vi "State_Machine.vi"(8 "error in (no error)":errorcluster caption="entrée d'erreur (pas d'erreur)", 11 "Wait_CloseFixture en entrée":refnum<class "Put_Weight.lvclass">) -> (0 "error out":errorcluster caption="sortie d'erreur", 2 "Json_String":string, 3 "Wait_CloseFixture en sortie":refnum<class "Put_Weight.lvclass">)   [LabVIEW 2020, in "Library Test.lvlib" / "Put_Weight.lvclass"]
uses:
  Put_Weight.lvclass
  C:/Users/ngarcin/OneDrive - Altyor/Standard TB/Class/Test/Test (Default)/Test (Default).lvclass
  Instrument/Instrument (Default)/Class Instrument (Default).lvclass
  Popup/Class Popup WaitWeight/Class Popup WaitWeight.lvclass
  C:/Users/ngarcin/OneDrive - Altyor/Standard TB/Class/Popup/Class Popup Operator_Validation/Class Popup Operator_Validation (Default)/Class Popup Operator_Validation (Virtual).lvclass
  C:/Users/ngarcin/OneDrive - Altyor/Standard TB/Class/Popup/Class Popup (Main)/Class Popup (Main).lvclass
  Put_Weight.lvclass/Put_Weight.ctl
  Commun VI/Library Commun.lvlib
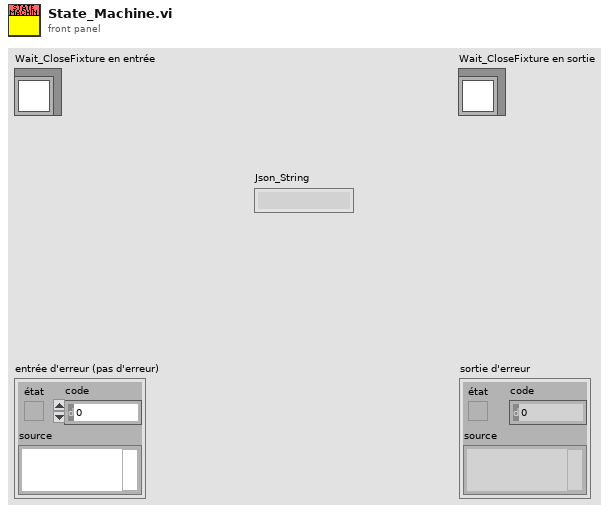
[diagram p1: front panel]
types:
  T1 = cluster{"Instrument":refnum<class "Class Instrument (Default).lvclass">, "Timeout (ms)":u64, "Weight":dbl, "Front":enum16{"Amount", "Descending"}}
  T2 = cluster{"Instrument DIO":refnum<class "Class Instrument (Default).lvclass">, "Valur for test":bool, "Timeout (ms)":u64}
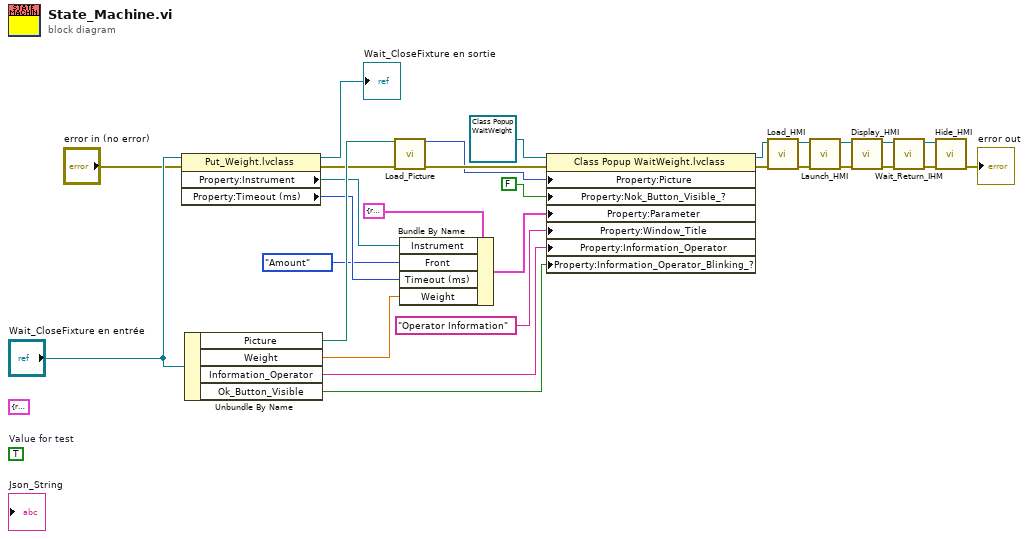
[diagram p0: block diagram]
diagram:
  (unwired) T2 {"Instrument DIO"=refnum, "Valur for test"=FALSE, "Timeout (ms)"=0} ("cluster")
  (unwired) TRUE  # Value for test
  n1 = property class="Put_Weight.lvclass"(reference="Wait_CloseFixture en entrée", error in="error in (no error)") -> (reference out=→"Wait_CloseFixture en sortie":refnum<class "Put_Weight.lvclass">, error out=w6:errorcluster, "Property:Instrument"=w8:refnum<class "Class Instrument (Default).lvclass">, "Property:Timeout (ms)"=w13:u64)
  n2 = Unbundle By Name("Wait_CloseFixture en entrée") -> ("Picture"=w21:path, "Weight"=w1:dbl, "Information_Operator"=w24:string, "Ok_Button_Visible"=w23:bool)
  n3 = call "Load_Picture.vi"("Chemin In"=w21, "error in (no error)"=w6) -> ("Img Out"=w20:picture, "error out"=w22:errorcluster)  [unwired: 11 in, 1 out]
  n4 = Bundle By Name(cluster=T1 {"Instrument"=refnum, "Timeout (ms)"=0, "Weight"=0.0, "Front"=enum."Descending"} ("Parameter"), "Instrument"=w8, "Front"=enum16{"Amount", "Descending"}."Amount", "Timeout (ms)"=w13, "Weight"=w1) -> (w5:T1)
  n5 = property class="Class Popup WaitWeight.lvclass"(reference=refnum<class "Class Popup WaitWeight.lvclass"> refnum ("Library Instrument & Equipement.lvlib:Library Popup.lvlib:Class Popup WaitWeight.lvclass"), error in=w22, "Property:Picture"=w20, "Property:Nok_Button_Visible_?"=FALSE ("Nok_Button_Visible_?"), "Property:Parameter"=w5, "Property:Window_Title"="Operator Information" ("Window_Title"), "Property:Information_Operator"=w24, "Property:Information_Operator_Blinking_?"=w23) -> (reference out=w28:refnum<class "Class Popup WaitWeight.lvclass">, error out=w27:errorcluster)
  n6 = call-dynamic "Load_HMI.vi"("error in (no error)"=w27, "Class Popup (Default) en entrée"=w28) -> ("error out"=w17:errorcluster, "Class Popup (Default) en sortie"=w18:refnum<class "Class Popup WaitWeight.lvclass">)  [unwired: 8 in]
  n7 = call-dynamic "Launch_HMI.vi"("error in (no error)"=w17, "Class Popup (Default) en entrée"=w18) -> ("error out"=w29:errorcluster, "Class Popup (Default) en sortie"=w19:refnum<class "Class Popup WaitWeight.lvclass">)  [unwired: 8 in]
  n8 = call-dynamic "Display_HMI.vi"("error in (no error)"=w29, "Class Popup (Default) en entrée"=w19) -> ("error out"=w12:errorcluster, "Class Popup (Default) en sortie"=w9:refnum<class "Class Popup WaitWeight.lvclass">)  [unwired: 8 in]
  n9 = call-dynamic "Wait_Return_IHM.vi"("error in (no error)"=w12, "Class Popup (Default) en entrée"=w9) -> ("error out"=w11:errorcluster, "Class Popup (Default) en sortie"=w10:refnum<class "Class Popup WaitWeight.lvclass">)  [unwired: 8 in]
  n10 = call-dynamic "Hide_HMI.vi"("error in (no error)"=w11, "Class Popup (Default) en entrée"=w10) -> ("error out"=→"error out":errorcluster)  [unwired: 8 in, 1 out]
